vi "Create Test Stations and Aliases.vi"(8 "error in":errorcluster) -> (0 "error out":errorcluster, 4 "log":string)   [LabVIEW 2024]
uses:
  <vilib>/Plug-In SDKs/Clients/Metadata/Test Station.ctl
  <vilib>/Plug-In SDKs/Clients/Metadata/Extension.ctl
  <vilib>/Plug-In SDKs/Clients/Metadata Store V1/Metadata Store Client.lvlibp/API/Metadata Store V1/Create Test Station.vi
  <vilib>/Plug-In SDKs/Clients/Metadata Store V1/Metadata Store Client.lvlibp/API/Metadata Store V1/Create Alias (Metadata - Test Station).vi
  <vilib>/Plug-In SDKs/Clients/Metadata Store V1/Metadata Store Client.lvlibp
  <vilib>/Plug-In SDKs/Clients/Metadata/NI Metadata Types.lvlib
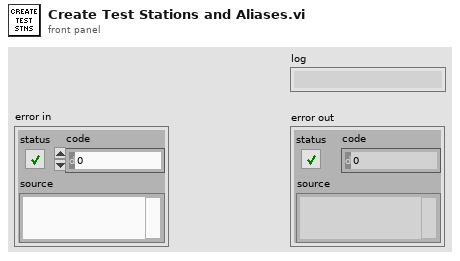
[diagram p1: front panel]
types:
  T1 = typedef "NI Metadata Types.lvlib/Test Station.ctl" = cluster{"name":string, "asset identifier":string, "id":string, "link":string, "extension":T2[], "schema id":string}
  T2 = typedef "NI Metadata Types.lvlib/Extension.ctl" = cluster{"name":string, "value":string}
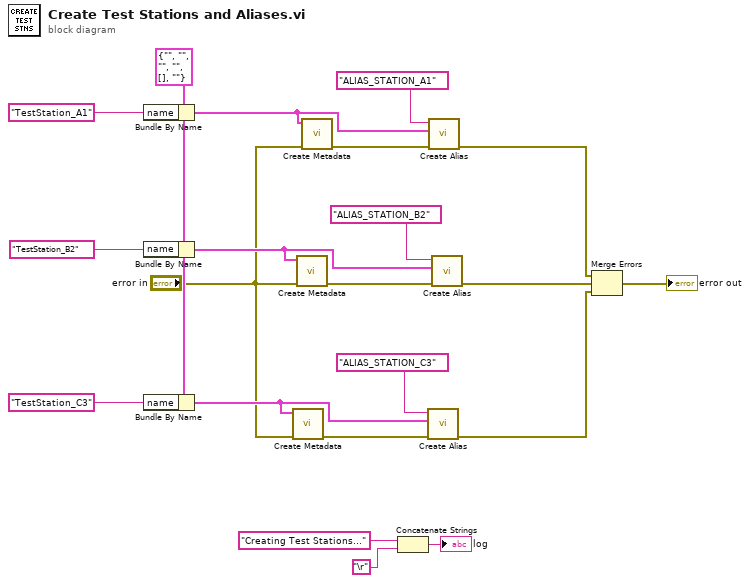
[diagram p0: block diagram]
diagram:
  w5 = T1 {"name"="", "asset identifier"="", "id"="", "link"="", "extension"=[], "schema id"=""} ("test station")
  n1 = Bundle By Name(cluster=w5, "name"="TestStation_A1" ("operator name")) -> (w12:T1)
  n2 = Bundle By Name(cluster=w5, "name"="TestStation_B2" ("operator name")) -> (w17:T1)
  n3 = Bundle By Name(cluster=w5, "name"="TestStation_C3" ("operator name")) -> (w16:T1)
  n4 = call-poly <vilib>:"Create Metadata.vi"("error in"="error in", "test station"=w16) -> ("error out"=w9:errorcluster)  [unwired: 8 in, 1 out]
  n5 = call-poly <vilib>:"Create Metadata.vi"("error in"="error in", "test station"=w17) -> ("error out"=w10:errorcluster)  [unwired: 8 in, 1 out]
  n6 = call-poly <vilib>:"Create Metadata.vi"("error in"="error in", "test station"=w12) -> ("error out"=w11:errorcluster)  [unwired: 8 in, 1 out]
  n7 = Concatenate Strings("Creating Test Stations..." ("role"), "\r") -> (→"log":string)
  n8 = call-poly <vilib>:"Create Alias.vi"("error in"=w9, "test station"=w16, "alias name"="ALIAS_STATION_C3") -> ("error out"=w20:errorcluster)  [unwired: 7 in, 1 out]
  n9 = call-poly <vilib>:"Create Alias.vi"("error in"=w11, "test station"=w12, "alias name"="ALIAS_STATION_A1") -> ("error out"=w18:errorcluster)  [unwired: 7 in, 1 out]
  n10 = call-poly <vilib>:"Create Alias.vi"("error in"=w10, "test station"=w17, "alias name"="ALIAS_STATION_B2") -> ("error out"=w19:errorcluster)  [unwired: 7 in, 1 out]
  n11 = Merge Errors(w18, w19, w20) -> (→"error out":errorcluster)
